vi "Do Recombination.vi"(8 "error in":errorcluster, 9 "IChromosome Parent B in":refnum<class "IChromosome.lvclass">, 10 "IChromosome Parent A in":refnum<class "IChromosome.lvclass">, 11 "N-Point Crossover in":refnum<class "N-Point Crossover.lvclass">) -> (0 "error out":errorcluster, 1 "IChromosome Child B out":refnum<class "IChromosome.lvclass">, 2 "IChromosome Child A out":refnum<class "IChromosome.lvclass">, 3 "N-Point Crossover out":refnum<class "N-Point Crossover.lvclass">)   [LabVIEW 2016, in "N-Point Crossover.lvclass"]
uses:
  N-Point Crossover.lvclass
  IChromosome/IChromosome.lvclass
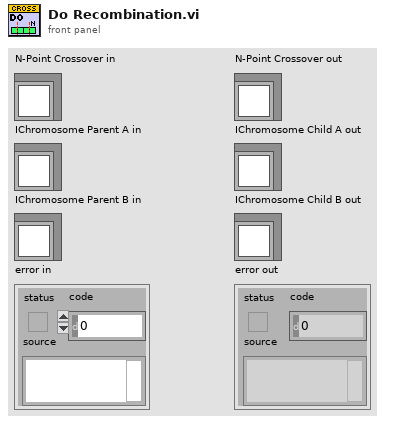
[diagram p1: front panel]
types:
  T1 = typedef "N-Point Crossover.lvclass/X-Point Crossover.ctl" = enum16{"Single-point Crossover", "Dual-point Crossover"}
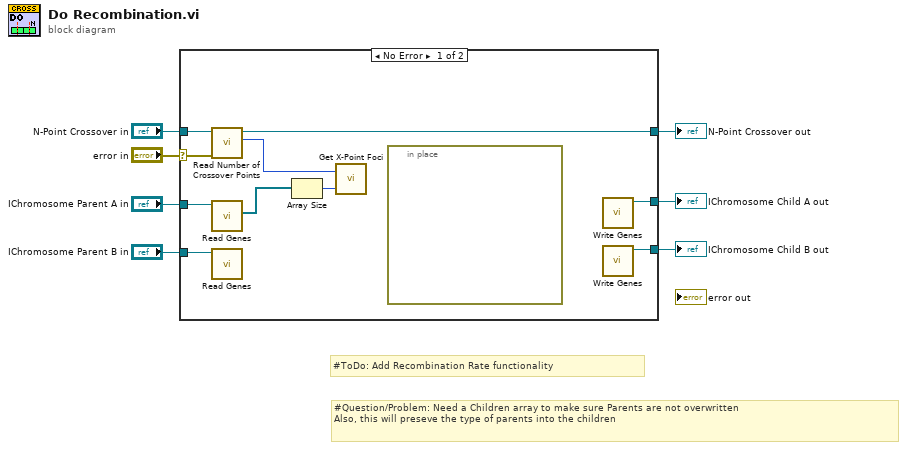
[diagram p0: block diagram]
diagram:
  # "#Question/Problem: Need a Children array to make sure Parents are not overwritten\nAlso, this will preseve the type of parents into the children"
  # "#ToDo: Add Recombination Rate functionality"
  n1 = case shown="No Error" "error in" {
    selector: "error in" -> [w15 _]
    tunnel: "N-Point Crossover in" -> [w17 w18]
    tunnel: [w16 w18] -> w5
    tunnel: "IChromosome Parent A in" -> [w14 _]
    tunnel: "IChromosome Parent B in" -> [w13 _]
    tunnel: [w9 _] -> w2
    tunnel: [w8 _] -> w1
    frame No Error {
      n2 = call "Read Number of Crossover Points.vi"("error in (no error)"=w15, "N-Point Crossover in"=w17) -> ("X-Point"=w11:T1, "N-Point Crossover out"=w16:refnum<class "N-Point Crossover.lvclass">)  [unwired: 7 in, 1 out]
      n3 = call "Read Genes.vi"("IChromosome in"=w14) -> ("Genes"=w12:refnum<class "IGene.lvclass">[])  [unwired: 8 in, 2 out]
      n4 = call "Read Genes.vi"("IChromosome in"=w13) -> ()  [unwired: 8 in, 3 out]
      n5 = Array Size(array=w12) -> (size(s)=w10:i32)
      n6 = call "Get X-Point Foci.vi"("Chromosome Length"=w10, "X-Point Type"=w11) -> ()  [unwired: 1 out]
      n7 = in-place {
      }
      n8 = call "Write Genes.vi"() -> ("IChromosome out"=w9:refnum<class "IChromosome.lvclass">)  [unwired: 10 in, 1 out]
      n9 = call "Write Genes.vi"() -> ("IChromosome out"=w8:refnum<class "IChromosome.lvclass">)  [unwired: 10 in, 1 out]
    }
    frame Error {
    }
  }
  "N-Point Crossover out" <- w5
  "IChromosome Child B out" <- w1
  "IChromosome Child A out" <- w2
